vi "ComputeBlocks.vi"(7 "SHA-1":refnum<class "SHA-1.lvclass">, 10 "blocks queue":refnum<queue>) -> (2 "hash":u8[](array[numeric]) format="%02x")   [LabVIEW 2013, in "SHA-1.lvlib" / "SHA-1.lvclass"]
doc: "This VI contains the core of the MD5 algorithm."
uses:
  SHA-1.lvclass
  Data-vector.ctl
  W-vector.ctl
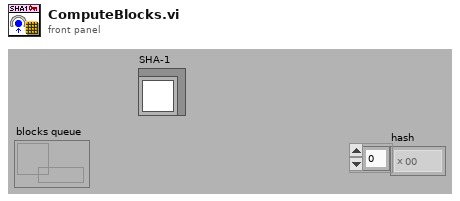
[diagram p1: front panel]
types:
  T1 = typedef "SHA-1.lvlib/SHA-1.lvclass/W-vector.ctl" = cluster{"W[80]":u32[], "end":bool}
  T2 = typedef "SHA-1.lvlib/SHA-1.lvclass/Data-vector.ctl" = cluster{"Data[ ]":u8[], "end":bool}
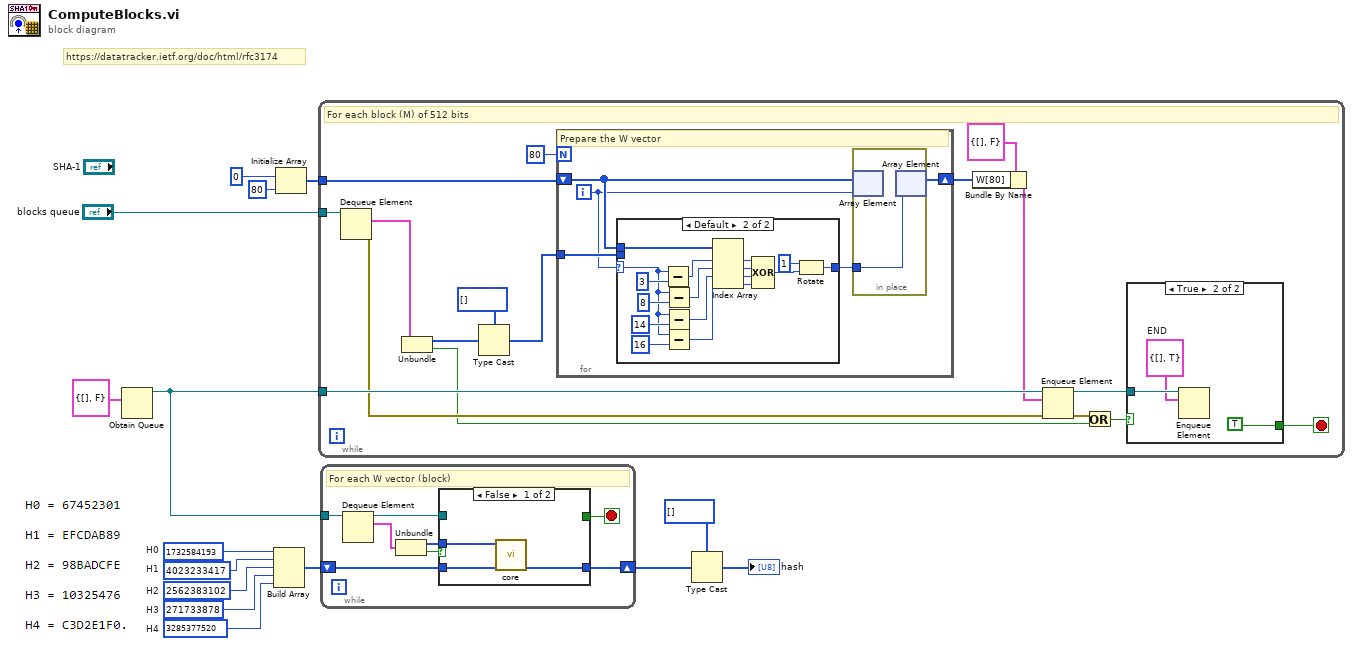
[diagram p0: block diagram]
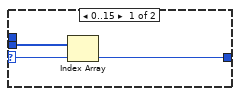
[diagram p3: hidden frame]
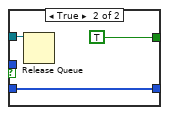
[diagram p4: hidden frame]
diagram:
  w10 = u32 3285377520  # H4
  w11 = u32 271733878  # H3
  w12 = u32 2562383102  # H2
  w13 = u32 4023233417  # H1
  w14 = u32 1732584193  # H0
  # "https://datatracker.ietf.org/doc/html/rfc3174"
  n1 = Obtain Queue(element data type=T1 {"W[80]"=[], "end"=FALSE} ("cluster")) -> (queue out=w6:refnum<queue>)  [unwired: 4 in, 2 out]
  n2 = Build Array(w14, w13, w12, w11, w10) -> (w8:u32[])
  n3 = Initialize Array(u32 0, 80) -> (w4:u32[])
  n4 = while {
    tunnel: "blocks queue" -> [w31]
    tunnel: w6 -> [w28]
    tunnel: w4 -> [w32]
    stop <- w16 stop-if-true
    # "For each block (M) of 512 bits"
    n5 = Dequeue Element(queue=w31) -> (element=w30:T2, error out=w20:errorcluster)  [unwired: 2 in, 2 out]
    n6 = Unbundle(w30) -> ("Data[ ]"=w29:u8[], "end"=w19:bool)
    n7 = Type Cast(type=u32[] [] ("U32"), x=w29) -> (*(type *) &x=w22:u32[])
    n8 = for {
      N: 80 -> [_]
      shift-right: [w39] -> w25
      shift-left: w32 -> [w37]
      tunnel: w22 -> [w40]
      i -> [w36]
      # "Prepare the W vector"
      n9 = case shown="Default" w36 {
        selector: w36 -> [w42 w57]
        tunnel: w40 -> [w44 _]
        tunnel: w37 -> [_ w45]
        tunnel: [w43 w46] -> w38
        frame 0..15 {
          n10 = Index Array(array=w44, index=w42) -> (element=w43:u32)
        }
        frame Default {
          n11 = Subtract(x=w57, y=3) -> (x-y=w52:i32)
          n12 = Subtract(x=w57, y=8) -> (x-y=w51:i32)
          n13 = Subtract(x=w57, y=14) -> (x-y=w50:i32)
          n14 = Subtract(x=w57, y=16) -> (x-y=w49:i32)
          n15 = Index Array(array=w45, index #1=w52, index #2=w51, index #3=w50, index #4=w49) -> (element #1=w56:u32, element #2=w55:u32, element #3=w54:u32, element #4=w53:u32)
          n16 = Compound Arithmetic op=XOR(w56, w55, w54, w53) -> (w47:u32)
          n17 = Rotate(1:w47, 2:i8 1 ("y")) -> (0:w46:u32)
        }
      }
      n18 = in-place {
        in-place-border: w38 -> [w41]
        n19 = in-place-array #1(w37, w36) -> ()  [unwired: 1 out]
        n20 = in-place-array #1(w41) -> (w39:u32[])  [unwired: 1 out]
      }
    }
    n21 = Bundle By Name(cluster=T1 {"W[80]"=[], "end"=FALSE}, "W[80]"=w25) -> (w23:T1)
    n22 = Enqueue Element(queue=w28, element=w23, error in (no error)=w20) -> (queue out=w21:refnum<queue>, error out=w18:errorcluster)  [unwired: 1 in, 1 out]
    n23 = Or(x=w18, y=w19) -> (x .or. y?=w17:bool)
    n24 = case shown="True" w17 {
      tunnel: w21 -> [_ w35]
      tunnel: [_ TRUE] -> w16
      frame False {
      }
      frame True {
        w34 = T1 {"W[80]"=[], "end"=TRUE}  # END
        n25 = Enqueue Element(queue=w35, element=w34) -> ()  [unwired: 2 in, 3 out]
      }
    }
  }
  n26 = while {
    shift-right: [w68] -> w7
    shift-left: w8 -> [w69]
    tunnel: w6 -> [w67]
    stop <- w62 stop-if-true
    # "For each W vector (block)"
    n27 = Dequeue Element(queue=w67) -> (queue out=w64:refnum<queue>, element=w66:T1)  [unwired: 2 in, 2 out]
    n28 = Unbundle(w66) -> ("W[80]"=w65:u32[], "end"=w63:bool)
    n29 = case shown="False" w63 {
      tunnel: w69 -> [w71 w75]
      tunnel: [w70 w75] -> w68
      tunnel: w65 -> [w72 _]
      tunnel: w64 -> [_ w74]
      tunnel: [_ TRUE] -> w62
      frame False {
        n30 = call "core.vi"("H[5] in"=w71, "W[80]"=w72) -> ("H[5] out"=w70:u32[])  [unwired: 9 in]
      }
      frame True {
        n31 = Release Queue(queue=w74) -> ()  [unwired: 2 in, 3 out]
      }
    }
  }
  n32 = Type Cast(type=u8[] [], x=w7) -> (*(type *) &x=→"hash":u8[])
